vi "testVideoCapture.vi"() -> ()   [LabVIEW 2024]
panel:
  in  "Length(s)":dbl=10.0 format="%#_13g"
  in  "SaveFile":string="DefaultMPegCodec"
  in  "Output Directory":path=path "E:/LTM Tests/VideoTests"
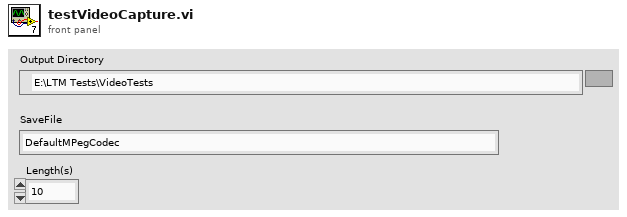
[diagram p1: front panel]
types:
  T1 = typedef "FFMpegRef.ctl" = cluster{"FFMpegRef":refnum<k24>, "StdOutRef":refnum<k24>, "DiagRef":refnum<k24>}
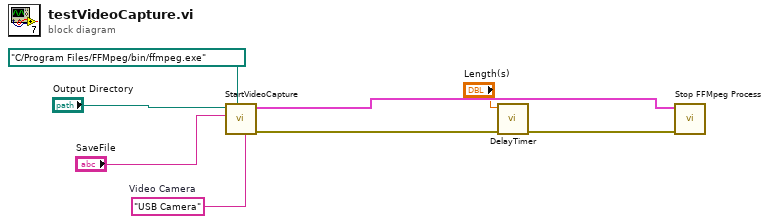
[diagram p0: block diagram]
diagram:
  w5 = "USB Camera"  # Video Camera
  n1 = call "StartVideoCapture.vi"("Output Directory"="Output Directory", "SaveFile"="SaveFile", "Path to FFMPEG"=path "C:/Program Files/FFMpeg/bin/ffmpeg.exe", "Video Camera"=w5) -> ("FFMpegProcess"=w2:T1, "error out"=w4:errorcluster)  [unwired: 5 in]
  n2 = call "DelayTimer.vi"("error in (no error)"=w4, "Delay(s)"="Length(s)") -> ("error out"=w3:errorcluster)  [unwired: 9 in]
  n3 = call "Stop FFMpeg Process.vi"("error in (no error)"=w3, "FFMpegProcess"=w2) -> ()  [unwired: 9 in, 1 out]
